vi "Estimate Maximum Step Size for LMS Adaptive Filter.vi"() -> ()   [LabVIEW 2019]
doc: "This example demonstrates how to estimate the maximum value of the step size for an adaptive filter that uses the LMS algorithm. By default, when you run this VI, this VI estimates the maximum step size for an adaptive filter and then uses that filter to identify the impulse response of an unknown system. You can analyze the accuracy of the filter by using the <b>Coefficients</b> graph.\n\nYou can manually override this estimation by clicking the <b>Use Estimated Step Size</b> button, entering a value for the <b>Step Size</b> control, and running the VI again. In this situation, the adaptive filter uses the step size you specify and not the estimated step size.\n\nThis example uses an FIR LMS adaptive filter to identify the impulse response of an unknown system. A lowpass FIR filter simulates the unknown system. The input to both this system and the adaptive filter is Gaussian white noise. The output of this system is the reference of the adaptive filter."
uses:
  <vilib>/addons/Adaptive Filters/Create/AFT Create FIR LMS (Real).vi
  <vilib>/addons/Adaptive Filters/Processing/AFT Filter Signal and Update Coefficients (Real, Array).vi
  <vilib>/addons/Adaptive Filters/Analysis/AFT Get Coefficients (FIR, Real).vi
  <vilib>/addons/Adaptive Filters/NI_AdaptiveFilter.lvlib
panel:
  in  "Use Estimated\nStep Size":bool=TRUE
  in  "Step Size":dbl=0.1 min=0.0 step=0.1
  out "Estimated Step Size":dbl
  in  "Filter Length":i32=25 min=2
  out "Coefficients":dbl[][](graph)
  out "Error Signal":dbl[](graph)
  # "Select Help>>Show Context Help and move the cursor over the VI icon of this example for more information."
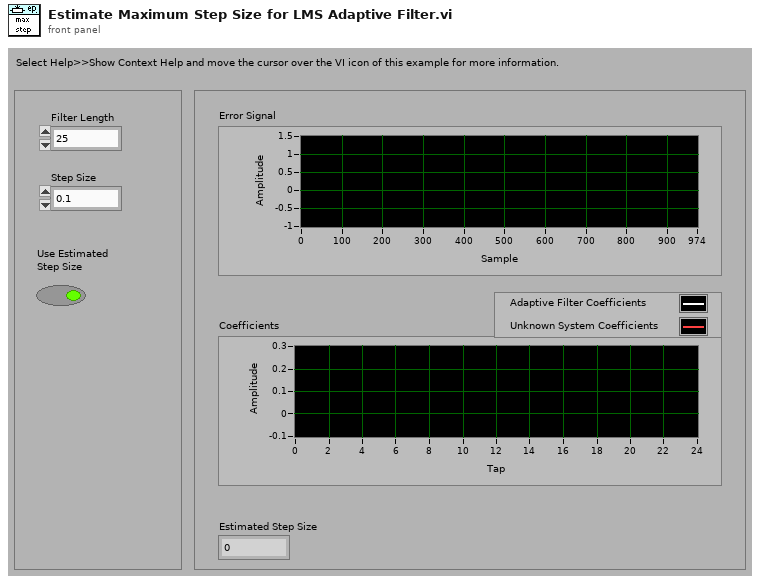
[diagram p1: front panel]
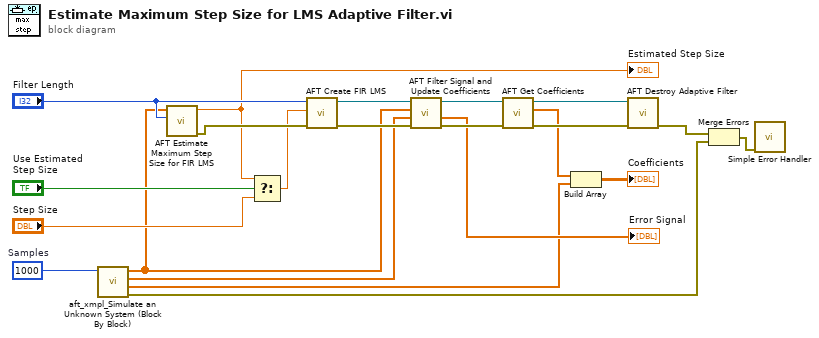
[diagram p0: block diagram]
diagram:
  w7 = 1000  # Samples
  n1 = call "aft_xmpl_Simulate an Unknown System (Block By Block).vi"("samples"=w7) -> ("error out"=w1:errorcluster, "unknown system coefficients"=w4:dbl[], "response signal"=w6:dbl[], "stimulus signal"=w5:dbl[])  [unwired: 3 in, 4 out]
  n2 = call <vilib>:"AFT Estimate Maximum Step Size for FIR LMS.vi"("filter length"="Filter Length", "x(n)"=w5) -> ("error out"=w12:errorcluster, "maximum step size"=w10:dbl)  [unwired: 1 in, 7 out]
  "Estimated Step Size" <- w10
  n3 = Select(t=w10, s="Use Estimated\nStep Size", f="Step Size") -> (s? t:f=w8:dbl)
  n4 = call-poly <vilib>:"AFT Create FIR LMS.vi"("error in (no error)"=w12, "step size"=w8, "filter length"="Filter Length") -> ("error out"=w21:errorcluster, "adaptive filter out"=w22:refnum<k20>)  [unwired: 1 in, 6 out]
  n5 = call-poly <vilib>:"AFT Filter Signal and Update Coefficients.vi"("error in (no error)"=w21, "d(n)"=w6, "x(n)"=w5, "adaptive filter in"=w22) -> ("error out"=w19:errorcluster, "e(n)"=→"Error Signal":dbl[], "adaptive filter out"=w20:refnum<k20>)  [unwired: 2 in, 3 out]
  n6 = call-poly <vilib>:"AFT Get Coefficients.vi"("error in (no error)"=w19, "adaptive filter in"=w20) -> ("error out"=w17:errorcluster, "coefficients"=w15:dbl[], "adaptive filter out"=w18:refnum<k20>)  [unwired: 7 out]
  n7 = Build Array(w15, w4) -> (→"Coefficients":dbl[][])
  n8 = call <vilib>:"AFT Destroy Adaptive Filter.vi"("error in (no error)"=w17, "adaptive filter in"=w18) -> ("error out"=w2:errorcluster)  [unwired: 9 out]
  n9 = Merge Errors(w2, w1) -> (w3:errorcluster)
  n10 = call <vilib>:"Simple Error Handler.vi"("error in (no error)"=w3) -> ()  [unwired: 1 in, 8 out]
